vi "Get Test Signal Configuration.vi"(11 "variant in":variant) -> (1 "signal configuration":refnum<class "SV Signal.lvclass">, 3 "variant out":variant)   [LabVIEW 2017]
uses:
  <vilib>/addons/_NISVFA/_Generation/Signal Generation/SV Signal/SV Signal.lvclass
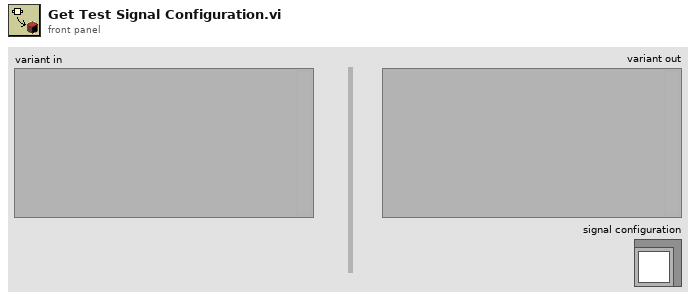
[diagram p1: front panel]
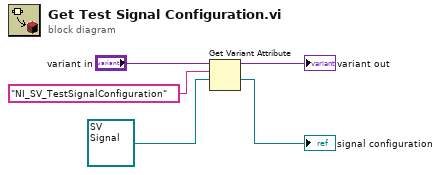
[diagram p0: block diagram]
diagram:
  n1 = Get Variant Attribute(Variant="variant in", name="NI_SV_TestSignalConfiguration", default value (empty Variant)=refnum<class "SV Signal.lvclass"> refnum ("dt [s]")) -> (duplicate Variant=→"variant out":variant, value=→"signal configuration":refnum<class "SV Signal.lvclass">)  [unwired: 1 in, 2 out]
